vi "Unflatten.vi"(8 "error in (no error)":errorcluster, 9 "timeout in":bool, 11 "CIFFifoCAN in":refnum<class "CIFFifoCAN.lvclass">) -> (0 "error out":errorcluster, 2 "Data":T2 {"payload" format="%x"; "identifier" format="%x"}, 3 "CIFFifoCAN out":refnum<class "CIFFifoCAN.lvclass">, 4 "Header":T1)   [LabVIEW 2021, in "CIFFifoCAN.lvclass"]
uses:
  CIFFifoCAN.lvclass
  ChannelRegistrar/typedef/Datatype CAN.ctl
  ChannelCommon/typedef/FIFO Header.ctl
  CIFFifoCAN.lvclass/CIFFifoCAN.ctl
  CIFFIFO/CIFfifo.lvclass/CIFfifo.ctl
  CIFFIFO/Accessors/Read Header.vi
  CIFFIFO/Accessors/Write Header.vi
  CIFFIFO/CIFfifo.lvclass
  ChannelCommon/ChannelCommon.lvlib
  ChannelRegistrar/ChannelRegistrar.lvlib
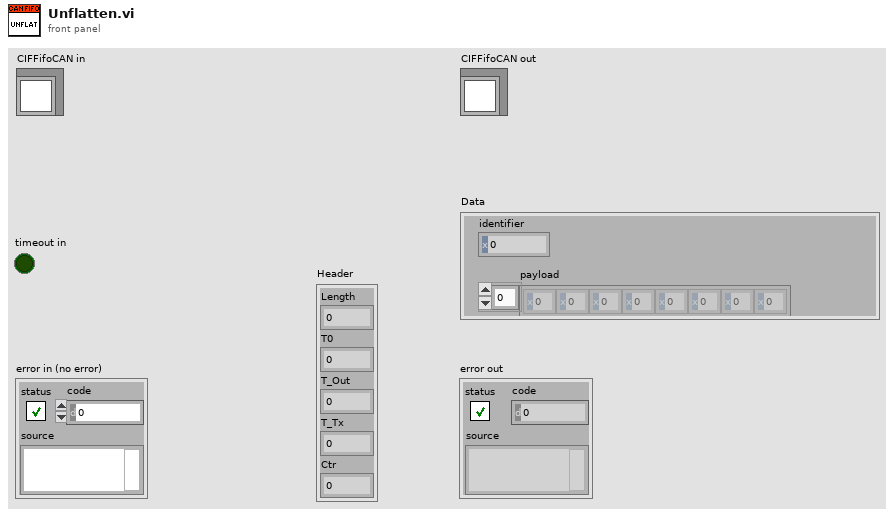
[diagram p1: front panel]
types:
  T1 = typedef "ChannelCommon.lvlib/FIFO Header.ctl" = cluster{"Length":u64, "T0":u64, "T_Out":u64, "T_Tx":u64, "Ctr":u64}
  T2 = typedef "ChannelRegistrar.lvlib/Datatype CAN.ctl" = cluster{"payload":u8[], "identifier":u32}
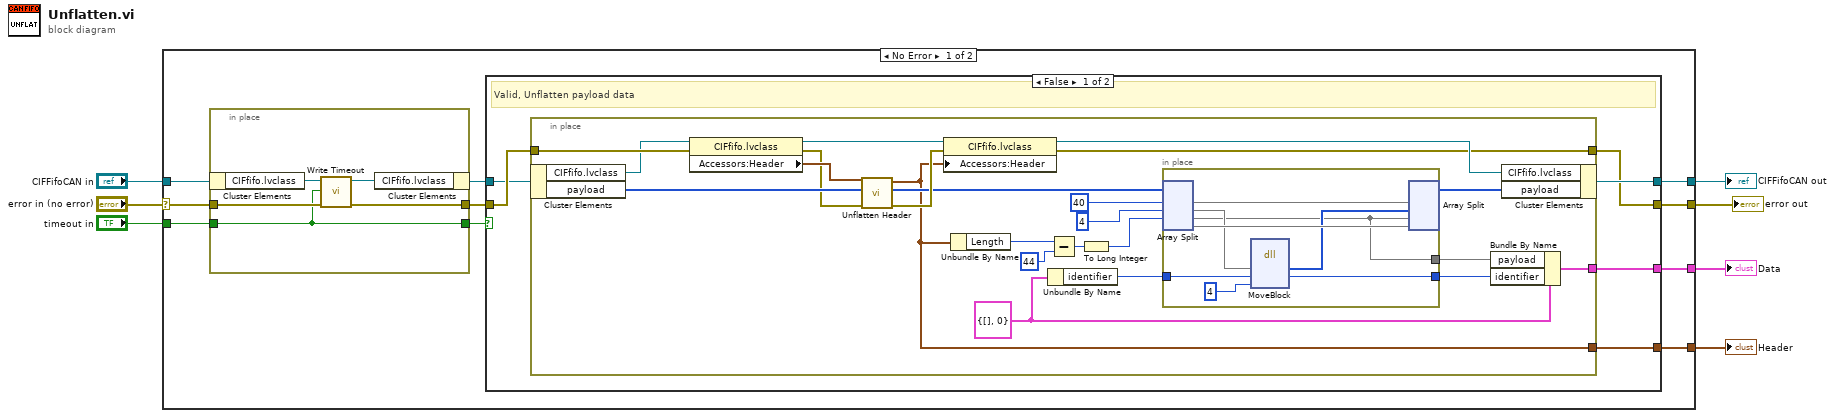
[diagram p0: block diagram]
diagram:
  n1 = case shown="No Error" "error in (no error)" {
    selector: "error in (no error)" -> [w16 w63]
    tunnel: [w9 w63] -> w6
    tunnel: [w10 w62] -> w4
    tunnel: "CIFFifoCAN in" -> [w17 w62]
    tunnel: "timeout in" -> [w15 _]
    tunnel: [w12 _] -> w2
    tunnel: [w11 _] -> w1
    frame No Error {
      n2 = in-place {
        in-place-border: w16 -> [w59]
        in-place-border: [w58] -> w14
        in-place-border: w15 -> [w57]
        in-place-border: [w57] -> w8
        n3 = in-place-cluster #1(w17) -> ("CIFfifo.lvclass"=w61:refnum<class "CIFfifo.lvclass">)
        n4 = call "Write Timeout.vi"("error in (no error)"=w59, "Timeout"=w57, "CIFFIFO in"=w61) -> ("error out"=w58:errorcluster, "CIFFIFO out"=w60:refnum<class "CIFfifo.lvclass">)  [unwired: 7 in]
        n5 = in-place-cluster #1("CIFfifo.lvclass"=w60) -> (w13:refnum<class "CIFFifoCAN.lvclass">)
      }
      n6 = case shown="False" w8 {
        tunnel: w14 -> [w23 w55]
        tunnel: w13 -> [w22 w56]
        tunnel: [w21 _] -> w12
        tunnel: [w20 _] -> w11
        tunnel: [w19 w56] -> w10
        tunnel: [w18 w55] -> w9
        frame False {
          # "Valid, Unflatten payload data"
          n7 = in-place {
            in-place-border: w23 -> [w45]
            in-place-border: [w27] -> w21
            in-place-border: [w26] -> w20
            in-place-border: [w25] -> w18
            w30 = T2 {"payload"=[], "identifier"=0} ("Data")
            n8 = in-place-cluster #2(w22) -> ("CIFfifo.lvclass"=w40:refnum<class "CIFfifo.lvclass">, "payload"=w46:u8[])
            n9 = property class="CIFfifo.lvclass"(reference=w40, error in=w45) -> (reference out=w42:refnum<class "CIFfifo.lvclass">, error out=w43:errorcluster, "Accessors:Header"=w44:T1)
            n10 = call "Unflatten Header.vi"("error in"=w43, "Flattened Data in"=w46, "Header in"=w44) -> ("error out"=w41:errorcluster, "Flatten Data out"=w38:u8[], "Header out"=w26:T1)  [unwired: 6 in]
            n11 = property class="CIFfifo.lvclass"(reference=w42, error in=w41, "Accessors:Header"=w26) -> (reference out=w39:refnum<class "CIFfifo.lvclass">, error out=w25:errorcluster)
            n12 = Unbundle By Name(w26) -> ("Length"=w35:u64)
            n13 = Unbundle By Name(w30) -> ("identifier"=w31:u32)
            n14 = Subtract(x=w35, y=u64 44) -> (x-y=w33:u64)
            n15 = To Long Integer(number=w33) -> (32bit integer=w32:i32)
            n16 = in-place {
              in-place-border: w31 -> [w51]
              in-place-border: [w48] -> w28
              in-place-border: [w47] -> w29
              n17 = in-place-split #3(w38, 40 ("y"), 4 ("y"), w32) -> (w54:u8[], w52:u8[], w47:u8[], w53:u8[])
              n18 = dll-call lib="LabVIEW" fn="MoveBlock"("source"=w52, "dest"=w51, "size"=u64 4) -> ("source"=w49:u8[], "dest"=w48:u32)  [unwired: 5 in, 2 out]
              n19 = in-place-split #3(w54, w49, w47, w53) -> (w24:u8[])  [unwired: 3 out]
            }
            n20 = Bundle By Name(cluster=w30, "payload"=w29, "identifier"=w28) -> (w27:T2)
            n21 = in-place-cluster #2("CIFfifo.lvclass"=w39, "payload"=w24) -> (w19:refnum<class "CIFFifoCAN.lvclass">)
          }
        }
        frame True {
          # "Timeout"
        }
      }
    }
    frame Error {
    }
  }
  "error out" <- w6
  "CIFFifoCAN out" <- w4
  "Data" <- w2
  "Header" <- w1
